vi "FlexibleBlock - Finite PCM Acquisition(Slave) - Left justified TI.vi"() -> ()   [LabVIEW 2021]
uses:
  <vilib>/PDM Acquisition Toolkit/host/Classes/Session/Controls/Logic Levels.ctl
  <vilib>/PDM Acquisition Toolkit/shared/controls/PCM Data Format Configuration.ctl
  <vilib>/PDM Acquisition Toolkit/shared/controls/Digital Edge.ctl
  <vilib>/PDM Acquisition Toolkit/shared/controls/PCM Bit Endianness.ctl
  <vilib>/PDM Acquisition Toolkit/shared/controls/PCM Data Justification.ctl
  <vilib>/PDM Acquisition Toolkit/shared/controls/PCM Frame Sync Control.ctl
  Program Files/National Instruments/LabVIEW 2021/examples/PDM Acquisition Toolkit/subVIs/PCM Interface Type.ctl
  Users/Admin/Desktop/Release audio branch/Audio/audio_d/audio_MeasurementService/source/measurements/ac/audio_acMeasurement/Measurement Results.ctl
  <vilib>/PDM Acquisition Toolkit/host/Classes/Tasks/PDM Tasks/Controls/Acquisition Mode.ctl
  <vilib>/addons/_NISVFA/_Shared subVIs/Controls/svc_Window.ctl
  <vilib>/addons/_NISVFA/_Shared subVIs/Common/SVL Set dB Reference (N Ch - 1 Ref).vi
  <vilib>/addons/Sound and Vibration/svt_Level/SVL AC & DC Level (Time) (N Ch).vi
  <vilib>/addons/Sound and Vibration/svt_Single Tone Measurements/SVT Spurious Free Dynamic Range (Frequency) (1 Ch).vi
  <vilib>/addons/_NISVFA/_Spectrum Processing/SVFA Unit Conversion (Complex) (1 Ch).vi
  <vilib>/addons/_NISVFA/_Shared subVIs/Common/SVL Set dB Reference (1 Ch).vi
  <vilib>/addons/Sound and Vibration/svt_Level/SVL AC & DC Level (Time) (1 Ch).vi
  <vilib>/addons/_NISVFA/_Spectrum Processing/SVFA Get Spectrum Subset.vi
  <vilib>/addons/_NISVFA/_Spectrum Processing/SVFA Get Spectrum Subset (Complex) (1 Ch).vi
  <vilib>/addons/_NISVFA/_Shared subVIs/Common/svc_Window Parameters.vi
  <vilib>/addons/_NISVFA/_Shared subVIs/Common/svc_Extract Single Tone Information (complex).vi
  <vilib>/addons/_NISVFA/_Shared subVIs/Common/svc_Check Frequency Range in Spectrum.vi
  <vilib>/addons/_NISVFA/_Spectrum Processing/SVFA Spectrum Peak Search.vi
  <vilib>/addons/_NISVFA/_Spectrum Processing/SVFA Spectrum Peak Search (1 Ch).vi
  <vilib>/addons/_NISVFA/_Shared subVIs/Common/svc_Spectrum Units.vi
  <vilib>/addons/_NISVFA/_Shared subVIs/Common/svc_Log View for Spectrum (1Ch).vi
  <vilib>/addons/_NISVFA/_Spectrum Processing/SVFA Unit Conversion (1 Ch).vi
  <vilib>/addons/_NISVFA/_Shared subVIs/Common/svc_Complex Datatype Defaults.vi
  <vilib>/addons/_NISVFA/_Shared subVIs/Common/svc_Build Unit Label for Frequency Range.vi
  <vilib>/addons/_NISVFA/_Shared subVIs/Common/SVL Set dB Reference (variant).vi
  <vilib>/addons/_NISVFA/_Shared subVIs/Common/svc_Get SV Channel Info.vi
  <vilib>/Analysis/baseanly.llb/Mean.vi
  <vilib>/Analysis/baseanly.llb/Mean (DBL).vi
  <vilib>/addons/_NISVFA/_Shared subVIs/Windowing/svfa_Scaled Time Domain Window (Array).vi
  <vilib>/addons/_NISVFA/_Spectrum Processing/SVFA Get Tone Amplitude and Phase (1 Ch).vi
  <vilib>/addons/_NISVFA/_Spectrum Processing/subVIs/svfa_Compute Complex Spectrum for Export.vi
  <vilib>/addons/_NISVFA/_Shared subVIs/Common/svc_Check Frequency Range in Bandwidth.vi
  <vilib>/addons/_NISVFA/_Shared subVIs/Common/svc_Convert Start and Stop to Start Index and Length.vi
  <vilib>/addons/_NISVFA/_Spectrum Processing/subVIs/svfa_Spectrum Peak Search.vi
  <vilib>/addons/_NISVFA/_Shared subVIs/Common/svc_Format Value (DBL).vi
  <vilib>/addons/_NISVFA/_Shared subVIs/Common/svc_Get Weighting Enum and Labels.vi
  <vilib>/addons/_NISVFA/_Shared subVIs/Common/svc_Engineering Units to Unit Label.vi
  <vilib>/addons/_NISVFA/_Shared subVIs/Common/svc_Surround NonAlpha String with Parentheses.vi
  <vilib>/dlg_ctls.llb/Space Constant.vi
  <vilib>/addons/_NISVFA/_Shared subVIs/Common/svc_Unwrap Phase.vi
  <vilib>/addons/_NISVFA/_Shared subVIs/Common/svc_Convert Spectrum Array to dB.vi
  <vilib>/addons/_NISVFA/_Spectrum Processing/subVIs/svfa_Conversion Utility (spectrum info).vi
  <vilib>/addons/_NISVFA/_Shared subVIs/Common/svc_Unit Label to Engineering Units.vi
  <vilib>/addons/_NISVFA/_Spectrum Processing/subVIs/svfa_Spectrum Info Window to windowTd Type Def.vi
  <vilib>/Analysis/4window.llb/Force Window.vi
  <vilib>/Analysis/4window.llb/Force Window (DBL).vi
  <vilib>/Analysis/4window.llb/Exponential Window.vi
  <vilib>/Analysis/4window.llb/Exponential Window (DBL).vi
  <vilib>/addons/_NISVFA/_Spectrum Processing/subVIs/svfa_Window Frequency Response.vi
  <vilib>/addons/_NISVFA/_Spectrum Processing/subVIs/svfa_Window Frequency Response (double array).vi
  <vilib>/Analysis/baseanly.llb/Dot Product.vi
  <vilib>/Analysis/baseanly.llb/Complex Dot Product.vi
  <vilib>/addons/_NISVFA/_Spectrum Processing/subVIs/svfa_Peak Rough Search Indices.vi
  <vilib>/addons/_NISVFA/_Shared subVIs/Common/svc_Unit Label Lexical Class.vi
  <vilib>/addons/_NISVFA/_Spectrum Processing/subVIs/svfa_Peak to RMS to Peak2Peak.vi
  <vilib>/addons/_NISVFA/_Spectrum Processing/subVIs/svfa_Mag to Mag2.vi
  <vilib>/addons/_NISVFA/_Spectrum Processing/subVIs/svfa_Linear to dB.vi
  <vilib>/addons/_NISVFA/_Spectrum Processing/subVIs/svfa_dBrefA to dBrefB.vi
  <vilib>/addons/_NISVFA/_Spectrum Processing/subVIs/svfa_Spectrum to Spectral Density.vi
  <vilib>/addons/_NISVFA/_Spectrum Processing/subVIs/svfa_Rect Window Frequency Response.vi
  <vilib>/addons/_NISVFA/_Spectrum Processing/subVIs/svfa_Cosine Window Coefficients.vi
  <vilib>/PDM Acquisition Toolkit/host/API/Public/Create Tasks/Create PCM Input Task.vi
  <vilib>/PDM Acquisition Toolkit/host/API/Public/Configure/Timing/Configure Timing - PCM Input Slave.vi
  <vilib>/PDM Acquisition Toolkit/host/API/Public/Configure/PDM Channel/Configure Microphone Sensitivity FSPA - PCM Input Task.vi
  <vilib>/PDM Acquisition Toolkit/host/API/Public/Utility/Configure Simulation Mode - PCM Input Task.vi
  <vilib>/PDM Acquisition Toolkit/host/API/Public/Start/Start PCM Input Task.vi
  <vilib>/PDM Acquisition Toolkit/host/API/Public/Read/Read PCM Input Waveform.vi
  <vilib>/measure/matone.llb/Extract Single Tone Information N Chan.vi
  <vilib>/PDM Acquisition Toolkit/host/API/Public/Clear/Clear PCM Input Task.vi
  <vilib>/addons/Sound and Vibration/svt_Weighting/SVT Weighting Filter (N Ch).vi
  <vilib>/addons/_NISVFA/_Shared subVIs/Common/svc_Caller VI Returned in Error Source.vi
  <vilib>/addons/_NISVFA/_Shared subVIs/Common/svc_Get Window Info.vi
  <vilib>/Analysis/0measdsp.llb/Scaled Time Domain Window.vi
  <vilib>/Analysis/0measdsp.llb/Scaled Time Domain Window (DBL).vi
  <vilib>/Utility/error.llb/Error Cluster From Error Code.vi
  <vilib>/Analysis/baseanly.llb/Std Deviation and Variance.vi
  <vilib>/addons/Sound and Vibration/svt_Single Tone Measurements/SVT Gain (Time) (1 Ch).vi
  <vilib>/addons/Sound and Vibration/svt_Distortion/SVT SNR without Harmonics (Frequency) (1 Ch).vi
  <vilib>/addons/Sound and Vibration/svt_Single Tone Measurements/SVT Dynamic Range (Frequency) (1 Ch).vi
  <vilib>/addons/Sound and Vibration/svt_Distortion/subVIs/sv_Check Data Valid (Audio) (1 Ch).vi
  <vilib>/addons/_NISVFA/_Shared subVIs/Common/svc_Convert Frequency to Frequency String.vi
  <vilib>/Analysis/4window.llb/window parameters.vi
  <vilib>/Analysis/4window.llb/Window Properties.vi
  <vilib>/Analysis/4window.llb/Window Properties by Name.vi
  <vilib>/addons/_NISVFA/_Spectrum Processing/subVIs/svfa_Spectrum Peak Tone Search and Estimation (complex).vi
  <vilib>/measure/masignal.llb/Tones and Noise Waveform.vi
  <vilib>/addons/_NISVFA/_Shared subVIs/Common/svc_FFT with Window.vi
  <vilib>/Analysis/1siggen.llb/Square Wave.vi
  <vilib>/addons/_NISVFA/_Spectrum Processing/subVIs/svfa_Three Finger Peak Search.vi
  <vilib>/addons/Sound and Vibration/svt_Distortion/subVIs/sv_Peak View Amplitude (1 Ch).vi
  <vilib>/PDM Acquisition Toolkit/host/API/PDM Acquisition Toolkit.lvlib
  <vilib>/PDM Acquisition Toolkit/host/Classes/Tasks/PDM Tasks/PDM Task.lvclass
  <vilib>/measure/NI_MAPro.lvlib
  <vilib>/PDM Acquisition Toolkit/shared/PDM Shared.lvlib
  <vilib>/addons/Sound and Vibration/svt_Single Tone Measurements/SoundVib_SingleTone.lvlib
  <vilib>/addons/Sound and Vibration/svt_Distortion/SoundVib_Distortion.lvlib
  <vilib>/addons/Sound and Vibration/svt_Weighting/SoundVib_ABCWeighting.lvlib
  <vilib>/PDM Acquisition Toolkit/host/Classes/Session/DecoderSession.lvclass
  Users/Admin/Desktop/Release audio branch/Audio/audio_d/audio_MeasurementService/source/measurements/ac/audio_acMeasurement/audio_acMeasurement.lvlib
panel:
  out "FreqDomainGraph":cluster{"x0":dbl, "dx":dbl, "magnitude":dbl[]}(graph) caption="AC"
  out "output cluster":T1
  out "error out 2":errorcluster
  in  "Latch Delay(ns)":sgl
  in  "PCM Interfaces":T2=enum."Left Justified"
  out "elements remaining":u32[](array[numeric])=[26]
  out "Frame Sync Clock Control":T3={"Frame Length"=64, "Frame Sync Pulse Width"=32, "Bit Clock Edge  Sync"=enum."Falling"}
  out "PCM Data Configuration":T5={"Frame Sync Edge for Channel 0"=enum."Falling", "Channel Count Per Frame"=2, "Channel Length"=32, "Bit Depth"=24, "Channel 0 Offset"=1, "Endianness"=enum."MSB First", "Data Justification"=enum."Left Justified"}
  in  "Bit clock rate":u32=12288000 format="%.4p"
  in  "logic level":T8
  out "Requested Sampling Rate":dbl=192000.0 format="%#_6p"
  out "detected phases (deg)":dbl[](array[numeric])=[48.77177137902379, 163.50683535190996] format="%.2p"
  out "detected amplitudes":dbl[](array[numeric])=[0.002127835538874218, 39.382575869286214] format="%.2p"
  out "detected frequencies":dbl[](array[numeric])=[87725.90443160792, 99.99819936214169] format="%.2p"
  in  "simulation mode":bool
  out "PCM Data":waveform(dbl)[](graph)=[{"t0"=timestamp(0 s since 1904-01-01), "dt"=5.208333277550992e-06, "Y"=array[4000 elements], "attributes"=variant("NI_ChannelName"=variant(string "PCMI0.0"))}, {"t0"=timestamp(0 s since 1904-01-01), "dt"=5.208333277550992e-06, "Y"=array[4000 elements], "attributes"=variant("NI_ChannelName"=variant(string "PCMI0.1"))}]
  in  "microphone sensitivity (dB/Pa)":dbl=0.34762
  in  "number of words":i32=19200
  in  "channel list":string="7820\\PCMi 0"
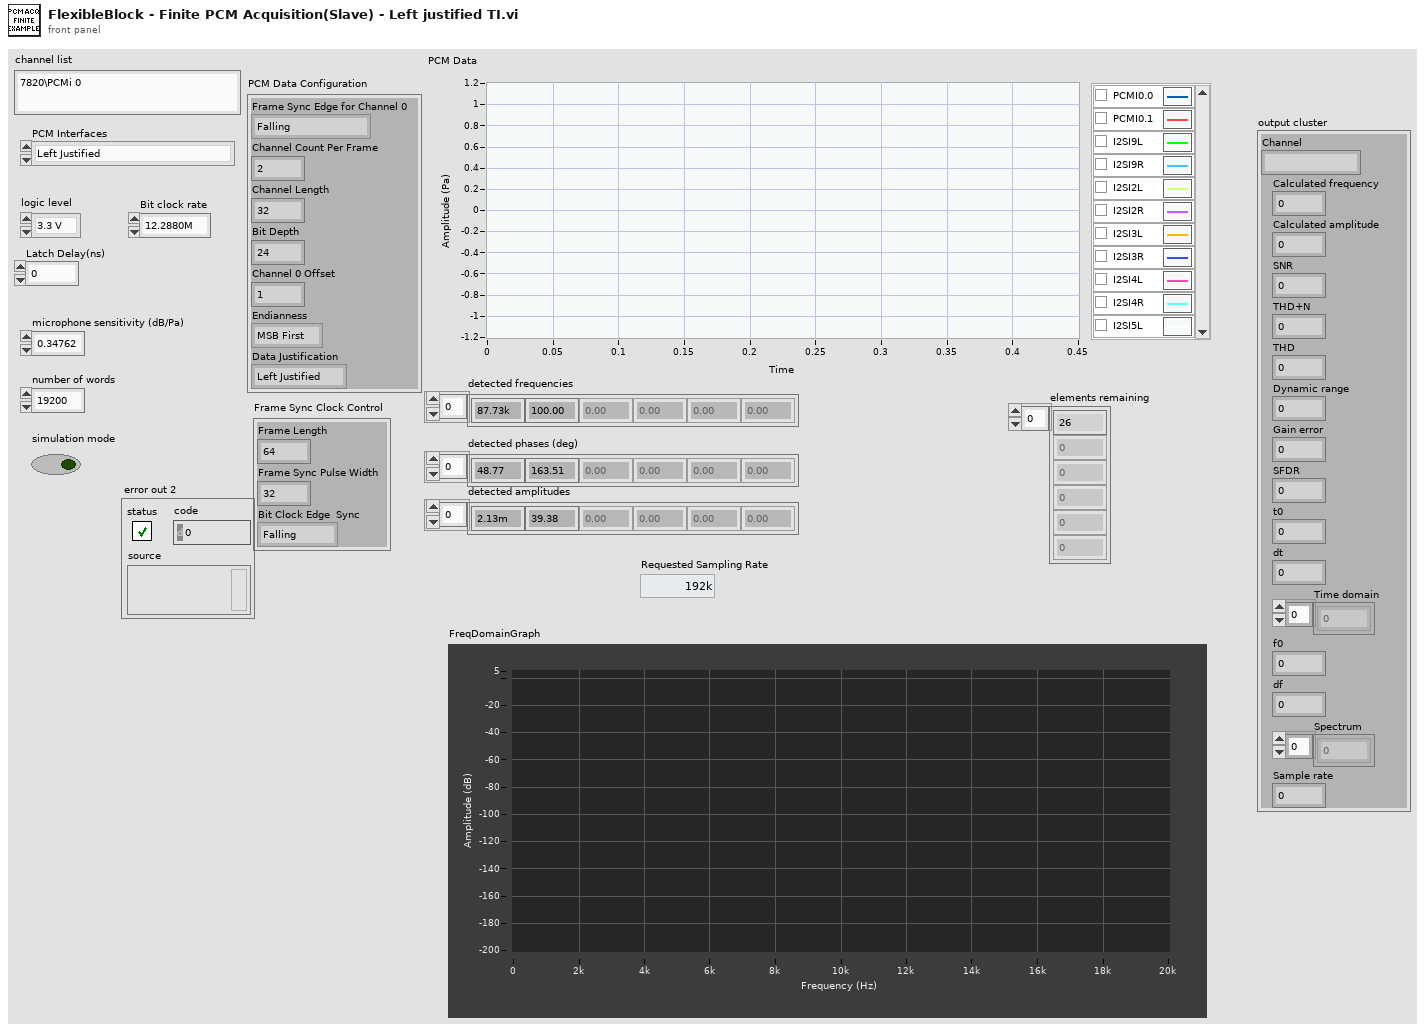
[diagram p1: front panel]
types:
  T1 = typedef "audio_acMeasurement.lvlib/Measurement Results.ctl" = cluster{"Channel":string, "Calculated frequency":dbl, "Calculated amplitude":dbl, "SNR":dbl, "THD+N":dbl, "THD":dbl, "Dynamic range":dbl, "Gain error":dbl, "SFDR":dbl, "t0":dbl, "dt":dbl, "Time domain":dbl[], "f0":dbl, "df":dbl, "Spectrum":dbl[], "Sample rate":u32}
  T2 = typedef "PCM Interface Type.ctl" = enum16{"I2S", "Left Justified", "Right Justified", "TDM 4 Channel", "TDM 6 Channel", "TDM 8 Channel", "DSP mode", "DSP mode with 1 bit delay", "PCM Short Frame", "PCM Long Frame"}
  T3 = typedef "PDM Shared.lvlib/PCM Frame Sync Control.ctl" = cluster{"Frame Length":u16, "Frame Sync Pulse Width":u16, "Bit Clock Edge  Sync":T4}
  T4 = typedef "PDM Shared.lvlib/Digital Edge.ctl" = enum8{"Rising", "Falling"}
  T5 = typedef "PDM Shared.lvlib/PCM Data Format Configuration.ctl" = cluster{"Frame Sync Edge for Channel 0":T4, "Channel Count Per Frame":u8, "Channel Length":u16, "Bit Depth":u8, "Channel 0 Offset":u16, "Endianness":T6, "Data Justification":T7}
  T6 = typedef "PDM Shared.lvlib/PCM Bit Endianness.ctl" = enum16{"MSB First", "LSB First"}
  T7 = typedef "PDM Shared.lvlib/PCM Data Justification.ctl" = enum16{"Left Justified", "Right Justified"}
  T8 = typedef "PDM Acquisition Class Library.lvlib/DecoderSession.lvclass/Logic Levels.ctl" = enum16{"3.3 V", "1.8 V", "1.2 V"}
  T9 = cluster{"Channel":string, "Calculated frequency":dbl, "Calculated amplitude":dbl, "SNR":dbl, "THD+N":dbl, "THD":dbl, "Dynamic range":dbl, "Gain error":dbl, "SFDR":dbl, "t0":dbl, "dt":dbl, "Time domain":dbl[], "f0":dbl, "df":dbl, "Spectrum":dbl[], "Sample rate":u32}
  T10 = cluster{"start frequency":dbl, "stop frequency":dbl}
  T11 = enum16{"no change", "spectrum", "spectral density"}
  T12 = cluster{"linear/dB":enum16{"no change", "linear", "dB"}, "dB reference (0: no change)":dbl, "power/magnitude":enum16{"no change", "power", "magnitude"}, "view":enum16{"no change", "rms", "peak", "peak-peak"}}
  T13 = cluster{"gain units":enum16{"dB", "linear ratio"}, "detected fundamental amplitude units":enum16{"EU rms", "EU peak", "EU peak-peak"}}
  T14 = typedef "svc_Window.ctl" = u32
  T15 = cluster{"SNR units":enum16{"dB", "linear ratio", "%"}, "detected fundamental amplitude units":enum16{"EU rms", "EU peak", "EU peak-peak"}}
  T16 = typedef "PDM Acquisition Class Library.lvlib/PDM Task.lvclass/Acquisition Mode.ctl" = enum16{"Finite", "Continuous"}
  T17 = typedef "PDM Acquisition Class Library.lvlib/PCM Input Task.lvclass/DVR PCM Input Task.ctl" = refnum<data-value>
  T18 = typedef "svc_Spectrum Info.ctl" = cluster{"channel name":string, "description":string, "x-axis units":T19, "spectral info":cluster{"spectrum type":T20, "linear/dB":enum16{"linear", "dB"}, "window":u16, "window size":i32, "FFT size":i32}, "engineering units":T21, "custom label":string, "dB reference [EU]":dbl, "peak units":enum16{"rms", "peak", "peak-peak"}, "weighting filter":T22, "spectral density?":bool, "unit label":string, "spectrum skewed?":bool, "complimentary spectrum units":T23}
  T19 = typedef "svc_X-Axis Units.ctl" = u16
  T20 = typedef "svc_Spectrum Type.ctl" = enum16{"FFT Spectrum [complex]", "Amplitude [Magnitude]", "Power [Magnitude^2]", "Cross Spectrum [complex]", "Frequency Response [Complex]"}
  T21 = typedef "svc_Engineering Units Text Ring.ctl" = u16
  T22 = typedef "svc_Weighting Filter Text Ring.ctl" = u16
  T23 = typedef "svc_Complimentary Spectrum Units.ctl" = enum16{"none", "radians", "degrees", "cycles", "imaginary"}
  T24 = cluster{"complex spectrum response":cluster{"f0":dbl, "df":dbl, "complex spectrum":cdb[]}, "spectrum info":T18}
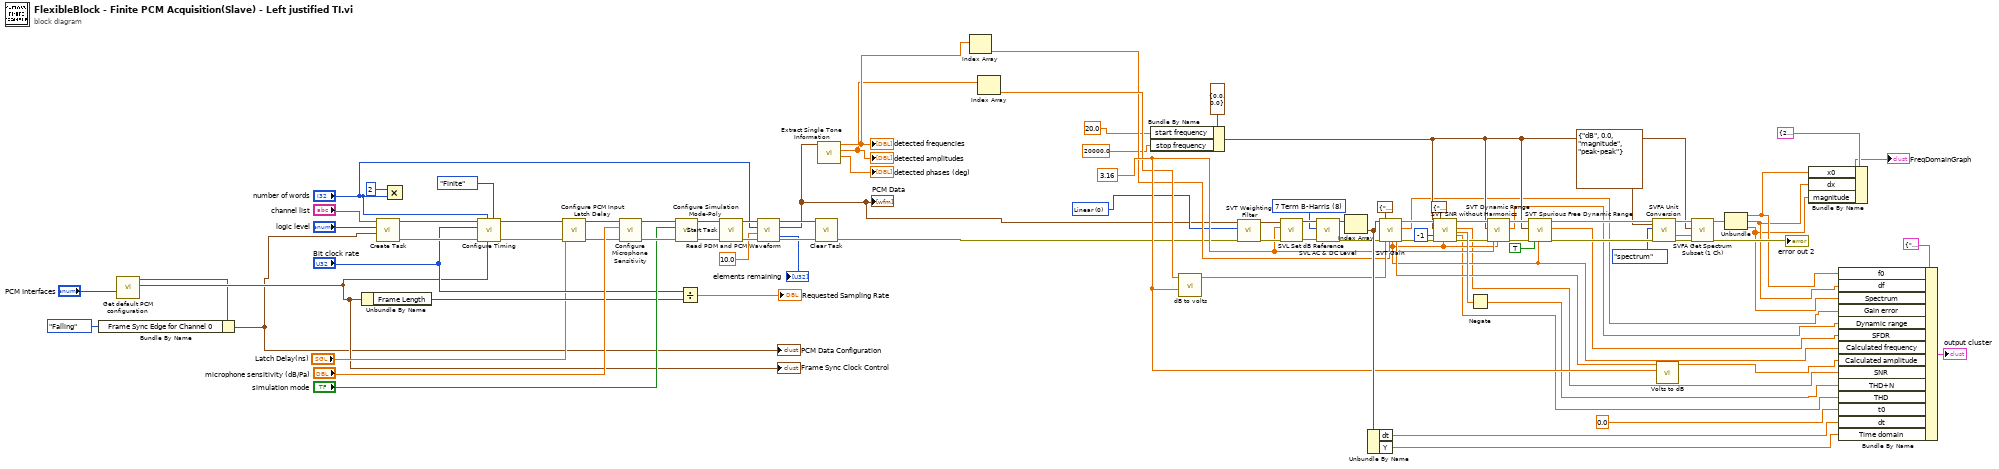
[diagram p0: block diagram]
diagram:
  w25 = u16 0 items=["Linear", "A-weighting", "B-weighting", "C-weighting"] ("weighting")
  w28 = 3.16 ("start frequency")
  w44 = T14 8 items=["None"=0, "Hanning"=1, "Hamming"=2, "Blackman-Harris"=3, "Exact Blackman"=4, "Blackman"=5, "Flat Top"=6, "4 Term B-Harris "=7, "7 Term B-Harris"=8, "Low Sidelobe"=9, "Force"=64, "Exponential"=65, "Blackman Nuttall"=11, "Triangle"=30, "Bartlett-Hanning"=31, "Bohman"=32, "Parzen"=33, "Welch"=34, "Kaiser"=60, "Dolph-Chebyshev"=61, "Gaussian"=62] ("window")
  n1 = call "Get default PCM configuration.vi"("PCM Interfaces"="PCM Interfaces") -> ("Frame Sync Clock Control"=w64:T3, "PCM Data Configuration"=w63:T5)  [unwired: 9 in]
  "Frame Sync Clock Control" <- w64
  n2 = Bundle By Name(cluster=w63, "Frame Sync Edge for Channel 0"=Digital_Edge."Falling") -> (w62:T5)
  "PCM Data Configuration" <- w62
  n3 = Unbundle By Name(w64) -> ("Frame Length"=w70:u16)
  n4 = call-poly <vilib>:"Create Task.vi"("PCM data configuration"=w62, "logic level"="logic level", "channel list"="channel list") -> ("error out"=w81:errorcluster, "PCM input task out"=w80:T17)  [unwired: 7 in]
  n5 = Multiply(x=2, y="number of words") -> ()  [unwired: 1 out]
  n6 = call-poly <vilib>:"Configure Timing.vi"("acquisition mode"=Acquisition_Mode."Finite", "Frame Sync Clock Control"=w64, "number of words per channel"="number of words", "error in"=w81, "Bit Clock rate"="Bit clock rate", "PCM input task in"=w80) -> ("error out"=w79:errorcluster, "PCM input task out"=w72:T17)  [unwired: 4 in]
  n7 = call <vilib>:"Configure PCM Input Latch Delay.vi"("error in"=w79, "Latch Delay(ns)"="Latch Delay(ns)", "PCM input task in"=w72) -> ("error out"=w78:errorcluster, "PCM input task out"=w77:T17)  [unwired: 6 in, 1 out]
  n8 = call-poly <vilib>:"Configure Microphone Sensitivity.vi"("error in"=w78, "microphone sensitivity (FS/Pa)"="microphone sensitivity (dB/Pa)", "PCM input task in"=w77) -> ("error out"=w85:errorcluster, "PCM input task out"=w84:T17)  [unwired: 7 in]
  n9 = call-poly <vilib>:"Configure Simulation Mode-Poly.vi"("error in"=w85, "simulation mode"="simulation mode", "PCM Input Task in"=w84) -> ("error out"=w75:errorcluster, "PCM Input Task out"=w76:T17)  [unwired: 7 in]
  n10 = Divide(x="Bit clock rate", y=w70) -> (x/y=→"Requested Sampling Rate":dbl)
  n11 = call-poly <vilib>:"Start Task.vi"("error in"=w75, "PCM input task in"=w76) -> ("error out"=w89:errorcluster, "PCM input task out"=w88:T17)  [unwired: 8 in]
  n12 = call-poly <vilib>:"Read PDM and PCM Waveform.vi"("error in"=w89, "timeout"=10.0, "words per channel"="number of words", "PCM input task In"=w88) -> ("error out"=w87:errorcluster, "PCM waveforms"=w8:waveform(dbl)[], "PCM input task out"=w86:T17, "elements remaining"=→"elements remaining":u32[])  [unwired: 4 in]
  "PCM Data" <- w8
  n13 = call-poly <vilib>:"Clear Task.vi"("error in"=w87, "PCM input task in"=w86) -> ("error out"=w9:errorcluster)  [unwired: 9 in]
  n14 = call-poly <vilib>:"Extract Single Tone Information.vi"("time signals in"=w8) -> ("detected phases (deg)"=→"detected phases (deg)":dbl[], "detected amplitudes"=w6:dbl[], "detected frequencies"=w7:dbl[])  [unwired: 5 in, 3 out]
  "detected frequencies" <- w7
  "detected amplitudes" <- w6
  n15 = Index Array(array=w7) -> (element=w26:dbl)  [unwired: 1 in]
  n16 = Index Array(array=w6) -> (element=w27:dbl)  [unwired: 1 in]
  n17 = Bundle By Name(cluster=T10 {"start frequency"=0.0, "stop frequency"=0.0} ("frequency range"), "start frequency"=20.0, "stop frequency"=20000.0 ("start frequency")) -> (w33:T10)
  n18 = call "dB to volts.vi"("Full scale range"=w28, "Voltage(dB)"=w27) -> ("Voltage(volts)"=w37:dbl)  [unwired: 9 in]
  n19 = call-poly <vilib>:"SVT Weighting Filter.vi"("error in (no error)"=w9, "weighting"=w25, "scaled signals [EU]"=w8) -> ("error out"=w58:errorcluster, "weighted signals [EU]"=w57:waveform(dbl)[])  [unwired: 6 in]
  n20 = call-poly <vilib>:"SVL Set dB Reference.vi"("error in (no error)"=w58, "dB reference [EU]"=w28, "scaled signals in [EU]"=w57) -> ("error out"=w45:errorcluster, "scaled signals out [EU]"=w47:waveform(dbl)[])  [unwired: 7 in]
  n21 = call-poly <vilib>:"SVL AC & DC Level.vi"("scaled signals in [EU]"=w47, "window"=w44, "error in (no error)"=w45) -> ("AC signals [EU]"=w46:waveform(dbl)[], "error out"=w53:errorcluster)  [unwired: 11 in, 4 out]
  n22 = Index Array(array=w46) -> (element=w60:waveform(dbl))  [unwired: 1 in]
  n23 = Unbundle By Name(w60) -> ("dt"=w15:dbl, "Y"=w14:dbl[])
  n24 = call-poly <vilib>:"SVT Gain.vi"("scaled signal [EU]"=w60, "error in (no error)"=w53, "desired units"=T13 {"gain units"=enum."dB", "detected fundamental amplitude units"=enum."EU peak"}, "amplitude [EU peak]"=w37, "expected fundamental frequency [Hz]"=w26) -> ("detected fundamental\nfrequency [Hz]"=w21:dbl, "detected fundamental\namplitude"=w36:dbl, "complex spectrum"=w42:T24, "gain"=w24:dbl, "error out"=w43:errorcluster)  [unwired: 9 in, 1 out]
  n25 = call-poly <vilib>:"SVT SNR without Harmonics.vi"("complex spectrum"=w42, "frequency range"=w33, "maximum harmonic"=-1, "error in (no error)"=w43, "desired units"=T15 {"SNR units"=enum."dB", "detected fundamental amplitude units"=enum."EU rms"}, "expected fundamental frequency [Hz]"=w21) -> ("complex spectrum"=w49:T24, "SNR (without harmonics)"=w19:dbl, "SINAD"=w50:dbl, "THD"=w17:dbl, "error out"=w48:errorcluster)  [unwired: 6 in, 3 out]
  n26 = Negate(x=w50) -> (-x=w18:dbl)
  n27 = call-poly <vilib>:"SVT Dynamic Range.vi"("complex spectrum"=w49, "frequency range"=w33, "error in (no error)"=w48, "full scale amplitude [EU peak]"=w28, "expected fundamental\nfrequency [Hz]"=w21) -> ("dup complex spectrum"=w54:T24, "dynamic range"=w23:dbl, "error out"=w55:errorcluster)  [unwired: 9 in, 3 out]
  n28 = call-poly <vilib>:"SVT Spurious Free Dynamic Range.vi"("complex spectrum"=w54, "frequency range"=w33, "error in (no error)"=w55, "exclude harmonics"=TRUE, "expected fundamental\nfrequency [Hz]"=w21) -> ("complex spectrum"=w40:T24, "spurious free dynamic range"=w22:dbl, "error out"=w41:errorcluster)  [unwired: 7 in, 5 out]
  n29 = call-poly <vilib>:"SVFA Unit Conversion.vi"("complex spectrum"=w40, "desired scaling"=T12 {"linear/dB"=enum."dB", "dB reference (0: no change)"=0.0, "power/magnitude"=enum."magnitude", "view"=enum."peak-peak"}, "spectral density desired"=T11."spectrum", "error in (no error)"=w41) -> ("converted spectrum"=w34:cluster{"x0":dbl, "dx":dbl, "magnitude":dbl[]}, "spectrum info out"=w30:T18, "error out"=w29:errorcluster)  [unwired: 10 in, 3 out]
  n30 = call "Volts to dB.vi"("Full scale range"=w28, "Voltage(V)"=w36) -> ("Voltage(dB)"=w20:dbl)  [unwired: 9 in]
  n31 = call <vilib>:"SVFA Get Spectrum Subset (1 Ch).vi"("spectrum"=w34, "range"=w33, "spectrum info"=w30, "error in (no error)"=w29) -> ("spectrum subset"=w32:cluster{"x0":dbl, "dx":dbl, "magnitude":dbl[]}, "error out"=→"error out 2":errorcluster)  [unwired: 10 in, 4 out]
  n32 = Unbundle(w32) -> ("x0"=w3:dbl, "dx"=w2:dbl, "magnitude"=w1:dbl[])
  n33 = Bundle By Name(cluster=cluster{"x0":dbl, "dx":dbl, "magnitude":dbl[]} {"x0"=20.000000214204196, "dx"=10.000000107102098, "magnitude"=[-114.15651603320237, -121.36305665533368, -143.37588801995145, -125.3747624869788, -122.11025021298603, -123.1180823220903, -136.70897783052968, -126.77027917479111, -124.020905313897, -126.88391294043589, -126.3843168978061, -126.4615231354403, -89.75481804806032, -54.76170840557006, -31.889535533022606, -16.187220558881673, -5.794808006347515, 0.16644842981875596, 2.111954876706231, 0.16568271315306057, -5.796393407051838, -16.18976327759025, -31.89341764484416, -54.76929643271966, -89.79463483193392, -125.27421120596713, -124.60058186076871, -123.95053059271027, -127.47180140959146, -139.09403229507976, -126.63006434840091, -121.07579620021035, -120.04129048879442, -123.47329398145577, -134.14891446501707, -146.20339758492725, -137.3896104617882, -126.31513036563122, -122.54359675626772, -122.43160900789394, -125.49078542917715, -130.19044820464535, -126.59317929836668, -124.64241946975281, -126.2021713620974, -128.1063542477712, -127.48703106495057, -125.76364372674362, -124.47688387334786, -125.23916835138252, -128.6971630825081, -136.56790005708194, -133.32615372072206, -131.72608576345402, -143.106858163413, -131.3095735071133, -124.29397195200927, -121.368674373711, -121.90246299165194, -128.19433975069393, -131.60782712391435, -126.8944252740466, -127.39742985708364, -127.71417117512829, -126.30679240498324, -125.19252731229923, -125.49993468715164, -126.39994800524063, -125.34042088344107, -124.67793859086814, -127.23965579624198, -135.84083632259842, -142.43150809477874, -134.0086167972518, -130.73012726416758, -130.1907568018264, -135.50609265421332, -133.4253285970364, -129.60229987874516, -131.13171834262775, -133.59386870323485, -135.71425492413542, -142.2170082364512, -136.95982490530557, -129.38136777852714, -127.98134492981278, -129.6797996357936, -130.20168657208524, -129.69250116743794, -132.18606004254426, -139.3365319883325, -142.95638009021565, -140.10103077135625, -137.90125131233873, -138.1172575189856, -137.12270326430053, -134.75157359049484, -131.036141399244, -129.58819028859088, -132.3121381683547, -132.23899142800224, -129.61404290235913, -131.74863783055739, -134.97852492231073, -130.67217091078922, -129.57964087194782, -130.57762641281138, -132.52834075522017, -135.78627621884178, -142.49901499322274, -141.48800399558812, -143.24757389814621, -136.19253726244997, -126.53142536309788, -123.34303583389666, -123.21233963987521, -124.41973762027126, -125.22134897615948, -126.9196904339552, -134.53612798046296, -131.3511435877546, -125.7114183660295, -126.40782929669791, -130.9162950852669, -131.9594582891918, -129.02418942942936, -127.10971294232291, -126.4224310677424, -126.82612865454529, -127.28676420603188, -126.88338795412825, -125.99706987988446, -125.40605453150732, -125.98578839299827, -127.64455962189358, -129.75927585242462, -133.09905622646616, -135.7466207774017, -134.00685547109643, -132.67495090714914, -132.22911014695032, -134.46516716691167, -132.93107087889965, -129.16213188426514, -128.36475477295505, -130.6578239989015, -139.01319588309485, -141.43076278882998, -132.5976905198517, -130.20172638885097, -131.94249777520935, -142.4683868052605, -137.91371427959592, -134.69530409837475, -139.30771283308204, -143.64947826069582, -132.63466050522175, -128.7962369961467, -128.39937836768866, -131.74873055308265, -138.6954450934956, -135.1962285419425, -132.09709522748193, -129.15949687453383, -126.11694756949157, -124.63202529768226, -124.94201741482676, -126.49196300473305, -128.6821678936123, -130.15958004607992, -130.1273796587127, -128.5745132662968, -128.1058374455199, -127.97528167034748, -126.56114707595619, -125.96083493714872, -128.04071224807072, -133.1177878962448, -133.10886671363295, -130.02517062749695, -127.71565199687112, -126.283155806085, -125.27620474949131, -124.43103341153218, -125.55086008570059, -127.69603922360118, -124.9973939221027, -123.63561955277645, -126.02696667962155, -131.0339686597125, -130.35947614827558, -128.56581326055817, -129.36696386233123, -131.51058997650355, -131.49345793307128, -130.2639756951258, -130.06154137992266, -131.30934831123636, -133.68725043425223, -131.21024897603903, -127.41427463637223, -126.56702895822193, -128.73574657204506, -135.2251528562724, -137.09878796045234, -129.65982047361766, -128.60824269595017, -133.9629685197531, -143.45429853804876, -133.13793023312388, -136.3576930963645, -140.18866650698027, -136.62431834777468, -149.51000061331155, -138.2575481284217, -135.40077239669253, -133.70402963095603, -129.62130848019223, -128.04003889661385, -129.07299362960455, -130.243010381597, -130.8356545145397, -134.25554995048782, -142.81225234393412, -143.35431562967096, -141.99768795418544, -133.72891879653776, -128.26376229949614, -126.4404753422564, -127.664694958722, -131.6546151781298, -133.9835508288192, -131.61025037102488, -129.76355892054818, -129.2146948095566, -130.47903981575715, -130.70294733784036, -127.96757949868831, -126.35288406579076, -126.31353409151642, -127.69465408451497, -130.10696674453473, -133.9953538092625, -138.95937651820464, -134.78023022337968, -133.40331646844584, -136.97210669828902, -137.6742245731884, -131.8935865116608, -128.08041416654765, -126.6030376158959, -129.1229728616486, -136.23524607274658, -137.99763315178393, -137.663888314118, -132.81444112514913, -128.94913192656026, -127.91873209867715, -128.83649192854074, -131.96946924832557, -140.50334657728865, -139.17357143500712, -130.04685541139634, -127.55399107211304, -128.5346865441011, -130.05619208428828, -131.5359224551727, -135.30272276609026, -140.56598466588264, -137.53864581132396, -135.36650264777796, -132.05021553801907, -127.08431322796868, -125.11638153620895, -126.51546380508822, -130.79487082356053, -135.8337500700424, -137.96789098268383, -137.6612174967581, -136.8525240136817, -137.89560180300387, -138.4163606363077, -138.89617197328573, -151.05555360581963, -140.0806379283803, -133.13438691626533, -130.67742331158985, -132.7009758726239, -137.7930300440105, -133.89079268203173, -132.3513933225086, -129.47466790985249, -128.675174172983, -134.2508781117415, -144.38217949112027, -143.25302137407414, -138.2432387296004, -133.18816048984561, -132.4476521016706, -132.27940648212274, -133.71593106085697, -130.97272419663955, -128.0071750015209, -128.32320844829786, -128.1322204714087, -126.11314825211852, -124.75764507735195, -125.00183660902866, -126.3881992622004, -126.68597521000366, -126.47721627454001, -128.63325217073626, -133.5154813873756, -133.6547303137009, -130.43733361296495, -127.71962150682313, -126.65473252724156, -128.18456744976507, -132.61617788973518, -138.6744162847475, -136.89280772607157, -131.05936965553266, -127.65982792402667, -127.61911554281396, -132.6356704141472, -145.5088139707351, -133.11481581885226, -129.8172964765464, -127.96031242256109, -127.1624773550662, -127.5334945461254, -128.77045709086252, -130.75805320448512, -133.73785033851098, -137.40393383108562, -140.64919530242383, -139.86263481002896, -139.27568424715585, -139.3165680812446, -136.37848592977173, -131.85564512858738, -128.04553654018565, -127.10046843375338, -127.70132337470984, -129.95972346253058, -136.15651152512513, -151.45234338455992, -136.34769248734867, -129.85335842932597, -125.62043839550992, -124.93110634255333, -127.2719922492762, -131.50099109954363, -134.24251753241893, -133.64061920992432, -135.34907730259997, -136.9361750228094, -139.4942004419679, -138.71830754900066, -131.35348239280097, -129.1847565855113, -128.93742401816604, -130.19230746987208, -132.7003727659455, -133.0516777985375, -130.97536944584454, -129.80754972375604, -130.85995618012333, -134.60541803793487, -144.58433965498182, -141.48074325063288, -133.1142287798377, -129.33650564449522, -126.52083915451094, -124.85767547811555, -125.039205853284, -125.76775672688633, -124.84425555853855, -123.0842008695624, -122.65967897754992, -124.43434703908707, -127.94012361622373, -132.03180970270643, -134.74422956385382, -134.1429029523909, -133.170624676105, -130.4381023904983, -128.38182637668285, -127.11788204516643, -126.09625608617152, -125.73095172423793, -126.56078991113168, -130.53076936926968, -147.6711161082625, -134.73874285097045, -132.45010923546954, -139.20610994728972, -144.12038561407957, -139.2934665775726, -133.33941953498666, -133.87196938118532, -137.92251592965744, -134.54376376378838, -135.10465774938206, -138.00036784453525, -140.14923829069366, -140.73594612300715, -135.31978861803103, -137.74981196351, -138.26679599379776, -130.02808759228776, -128.26232136313172, -129.5641718920475, -132.19935058576607, -136.61513212940693, -137.70405663224665, -132.94970694747306, -131.44414608568366, -131.39825444499925, -129.0592354923359, -126.77224109121286, -126.35431094572881, -127.11920218331377, -128.1590380561889, -132.54602468036273, -147.4097457828696, -132.66405562662808, -130.71098010220967, -131.13083905442704, -134.78108336536906, -144.53443589755935, -135.07906733275942, -131.00735560209276, -129.39549573091338, -130.94279831223741, -135.41063782985458, -139.89715600727968, -136.8353301788793, -133.1637671688385, -132.53876951223558, -135.86101805382629, -133.90049747804736, -129.27812427844404, -127.35043485949639, -126.70321117078687, -127.45904928107025, -129.31783333493055, -129.92679474398406, -129.27971386920967, -130.00018536685386, -128.9859740832338, -127.74720161522279, -131.35885053377064, -148.81785299198384, -135.1841137130214, -131.30044601743242, -130.2603569676074, -130.8089224292011, -132.2498404542057, -133.65829608602294, -135.33263985349686, -131.89623349713796, -127.83325622000918, -127.22791275050872, -129.57278397746532, -133.40149275610327, -134.0800544187885, -131.9310482478005, -132.35412217024768, -138.58371220502386, -131.04898036877447, -126.62984506457768, -125.65832818838884, -126.79449295419846, -129.1989464618408, -128.89501813476937, -127.71055226666991, -128.35201039176778, -128.78196491305584, -127.67883831390327, -126.61656217913246, -127.21217342691894, -128.53623925730813, -127.68098815225079, -127.88852615448995, -128.4140889308591, -127.15131844869303, -125.61051516912214, -124.43626065305368, -125.2051776368406, -129.521146725487, -136.46092559983086, -133.9930073209309, -133.4073275429007, -144.590380697332, -134.34271862706476, -129.57012341874486, -130.00992420856122, -133.73251748553523, -141.5502231794172, -140.04976832277276, -134.5079774386407, -131.67807173506742, -130.4172360660502, -129.42565663046753, -128.92218492602433, -130.59264886399205, -133.7369795995416, -130.41321499027114, -128.31516713641906, -130.24025121906206, -137.12637454195058, -145.21921974900937, -134.7715825912015, -131.23532439184356, -130.2829285815037, -129.7996696612736, -131.59985598104026, -137.39979799305587, -145.93688668306794, -137.00808684890555, -130.6964697519213, -128.99477114198365, -129.31059962430828, -129.1301276791428, -128.50071981657925, -127.88315655628146, -126.46125341801414, -125.53895633397144, -126.10664095039637, -128.57319122135647, -129.87075018141476, -129.64489172570515, -132.56487087993452, -141.6528124552129, -139.24493094304057, -131.8661976364603, -129.48357920444943, -128.838194919264, -128.86696820719897, -129.1182549107291, -129.276752155319, -130.50307398251564, -131.99953643570313, -133.23539632489323, -138.4905558435136, -137.08561310159223, -131.39620717185255, -129.2081990042275, -129.10928031059265, -131.22866296683628, -132.52532548394962, -129.16741984258266, -127.162610480911, -129.75500709172277, -138.05884875708298, -132.22950034834076, -128.98504167735345, -126.62201834882076, -126.60869755269948, -129.88482749687927, -136.36335481024477, -136.13049587489897, -133.8884618323441, -130.84390588685744, -127.09543624684672, -126.45898289944327, -130.26337052071307, -132.27768221924157, -126.69271310562154, -124.77324115553408, -125.07700001103174, -126.39423779383688, -128.45690525550663, -132.88581266275648, -141.63160035134737, -131.6789666347667, -128.17411609759813, -127.86393006040691, -129.09857776095288, -130.37683399418086, -130.48857325472878, -131.97120435437375, -132.17255321428806, -128.82835770307037, -125.51831606305548, -123.74257230980672, -124.01121775813436, -127.3178662591301, -135.66201835184535, -132.2764362005697, -127.88921506195166, -126.49793506836055, -126.54317231546797, -128.28991369920078, -132.28041101886913, -134.36951957288161, -131.12640145365083, -130.53958667504926, -133.19516620998962, -140.0012901923717, -141.94929210952708, -136.07051703087043, -136.97684034414075, -140.00144181656984, -138.21612577381376, -140.76837369696437, -135.97989944881246, -133.01488465136433, -135.74568686311724, -138.4317533132987, -133.699313169655, -132.4857861537641, -131.70064319055524, -129.52009624293703, -127.02717936923707, -126.13225053347067, -127.68835165412906, -131.28683149164067, -132.793748900352, -133.70138952533594, -133.8150620263195, -130.51346391520588, -128.84985757832328, -127.68718694870275, -126.13638519540808, -125.27597045706825, -125.12895012765941, -125.20089966751287, -125.96008249177302, -128.0865349903974, -131.10087328748972, -134.75057982525985, -133.75328927395412, -130.45539097090005, -131.3194658841701, -141.90359796485697, -132.31741787919046, -126.8976040873404, -127.09010857421609, -131.01364642141783, -132.5608588172204, -133.1003527631429, -133.29649981808484, -129.55841592288726, -128.72567394837557, -132.45273358509388, -149.84866149457767, -137.67276113570475, -135.37470909323818, -140.12502387674152, -140.65755931138963, -130.09019903413676, -125.31903068060751, -123.44159833636911, -124.07844165525175, -126.27532781551463, -128.11698626517995, -129.93503279161055, -131.00534012754505, -130.16009147564688, -129.71748332913967, -131.20476346088725, -135.0606166107994, -138.21203916558733, -132.7377616824591, -129.9345422966717, -128.54500865501154, -127.00241898048121, -126.22443434895482, -126.61490509228963, -127.56257611580777, -129.39942205378213, -134.03174882812462, -135.55004397449244, -129.9464625852486, -127.00529096573051, -126.34429137874328, -127.802644811231, -129.71233311779847, -130.77955552504602, -134.11824341731727, -145.29073872325128, -130.86874952497348, -126.49219125362087, -125.51681287261788, -126.67449358683199, -129.02771456133084, -129.3818490067665, -128.51134286587535, -128.35620607495213, -128.11722401348587, -128.3130759548645, -129.99536595996952, -132.29064435013981, -130.70414529104724, -127.10006059467828, -125.70174942765972, -126.85029458207892, -130.05831133701048, -133.94553912926082, -140.0791993172447, -137.2780369565474, -133.1110770272686, -130.59818142231066, -126.9481921470033, -125.42892293135063, -125.4687758796935, -127.1641244302916, -132.98222674979925, -138.9734289321744, -131.49285227286728, -128.7694265812654, -127.73023640566508, -129.26444713524572, -135.16014944866103, -134.92392269671907, -132.9869975924077, -132.6795931101827, -132.04575219482038, -131.06532995620464, -129.8050719377489, -128.7406509520967, -130.3111202664169, -141.7229618143493, -132.8277450492622, -130.21071064893025, -134.62590313714688, -147.6384379221752, -138.7819109391997, -135.52537884096105, -141.51928967709938, -139.4185570167782, -137.57557999929907, -139.54572045143098, -137.68651212869054, -133.9467959834045, -134.1604389388604, -138.55688137983648, -131.525531225989, -127.22042353812448, -126.98616874013584, -129.3992002956473, -133.3532631917223, -133.70540902612575, -128.00339883058052, -125.39409563073635, -126.21233400228485, -128.75457392554503, -127.07712950709366, -126.11135063391721, -128.79979095374705, -133.70129910129313, -133.39740602632497, -132.31882383172749, -133.70939703773558, -137.90095688770901, -137.702406748392, -132.81796747938506, -130.18046750876536, -130.60775525183064, -132.62311309117305, -133.34982444438825, -133.5130876057437, -132.08906184840237, -129.8330907049975, -129.58934674394956, -130.7793666265536, -129.3312651115063, -129.00815038846991, -131.7868493277033, -136.15506251920868, -136.58953561343742, -136.98648329762946, -156.09154258422765, -136.3993207154312, -133.99911977430864, -134.5342642454817, -131.64377042290658, -129.28528970315546, -130.73713871730166, -138.1450242269703, -143.12771377142388, -135.5095193027515, -133.2827418379652, -133.78200524612797, -128.90434266259803, -125.47905925595104, -124.7851928330207, -126.98439231485304, -132.9594053683025, -136.9240663579998, -129.9024175644099, -125.317739570323, -123.6267210650635, -124.43267769156253, -127.37067687006046, -129.41517108910898, -129.20164631430853, -128.86899661862498, -128.11815230821324, -128.2115034976673, -129.53942198882626, -132.53444686451263, -143.4477692136308, -136.67568534681155, -130.90682944841578, -130.258104371618, -133.06896289787474, -145.39868164901216, -138.53183084544116, -134.50980778823376, -136.85875097828932, -140.61844640654363, -140.31205962196015, -133.8107222956887, -130.6110971462344, -131.87976429464007, -144.90403424309747, -132.20039505502632, -128.12507401300797, -129.71060822762783, -134.53859155226854, -134.73000777271366, -132.4609126111234, -132.29226702211295, -136.57800600993187, -151.1682586912211, -133.83977180579947, -130.0678401903246, -128.31600061089776, -127.08026292808452, -127.03493167845112, -127.45866969454404, -127.68676320629547, -129.09762856777132, -132.15364089986218, -134.04115428087206, -133.8779411464501, -132.0940499376788, -129.8350963346672, -128.85792307464442, -129.61110586568043, -130.96617607036728, -130.88154107532247, -129.28705567428938, -127.95609325559181, -127.50898840016848, -129.23559386268602, -134.04225947473645, -131.1340523000352, -130.92571209032178, -128.5602479879214, -125.6871345118046, -125.11912389362051, -126.24048123990843, -129.24535806163271, -132.5440886995646, -132.9954683362444, -136.12535515056248, -143.1618213572715, -133.94450536877093, -132.89376396921097, -129.6896132256777, -126.08767480217482, -124.78131242391572, -124.2630312563219, -124.11882131678357, -125.21905062996382, -128.20274801786485, -132.94546383836746, -134.2290453348339, -131.32176658377392, -129.71928378439375, -129.42446020016828, -129.8796130717054, -128.27635658130194, -128.42269621026605, -132.82075551623282, -136.1775161268704, -134.83166284300924, -130.91110156090878, -129.7226134122634, -131.44403452385663, -132.2830567724897, -129.7998097743775, -127.18084830701955, -125.85332351640282, -125.94019803617533, -127.12682941085392, -128.61695475350868, -129.7573076554893, -131.73105506979473, -136.52115876021065, -145.25392676654616, -154.40045789778497, -140.80592093742683, -133.8405262954971, -131.4216771987439, -132.78047100476175, -135.54634408756104, -135.95641648009197, -133.46076477633687, -133.3282158920459, -138.77983737457188, -146.53613685792283, -137.25006501914305, -131.0624241972309, -125.61996667947193, -122.73337965201776, -122.6992563957289, -125.0977045208799, -129.65788815938575, -133.85348282371456, -131.29842539900136, -132.32702770596177, -134.27326435823292, -129.1828971170441, -127.53331466556858, -128.04572023790135, -129.4051778201533, -129.12273514934617, -126.82476073177594, -126.7554523871324, -130.05646045486446, -133.12963431707558, -133.70846963996232, -133.5223055372282, -131.68011905188928, -129.97896879557206, -129.53502168992873, -131.03289102472633, -129.29673198034163, -126.46010756079349, -127.21270133997794, -131.69357233781957, -141.17552753342542, -136.92832494872553, -132.38809330970864, -129.99887465693874, -130.20986732760488, -133.24353656356416, -133.84431973429733, -131.92935389324722, -133.42639065281716, -151.35973915724958, -128.82271027063123, -124.41826711809475, -125.47774102219044, -133.53317624304682, -130.3583911258403, -124.85743487186735, -123.24232506273803, -123.76339290076822, -126.99586618548256, -134.3715325774083, -134.96014317682452, -135.35657690982578, -136.85181787996262, -129.80784607268754, -128.52967293150354, -131.41491565997063, -137.13644569463204, -142.48901007926804, -144.51871042193648, -145.09209018458304, -150.71861969534078, -135.16878599477513, -130.9569616252235, -131.03623501717556, -132.54770325374392, -134.4247607870267, -136.59539355594598, -137.52497886062497, -138.71558724297176, -138.41746910528656, -136.75402178489824, -137.21437189811726, -132.940815797596, -131.0676585481675, -131.5638283390021, -132.3066878366566, -131.2157643456185, -128.33466936681063, -125.23446374477857, -124.12297037494608, -125.29432052990711, -127.57046668571944, -128.26446586561138, -127.776321646176, -127.16152220808002, -127.35209371373928, -130.0907687167644, -135.6684518443326, -138.21315090732065, -152.4609447865921, -134.48178808548644, -130.01759392458277, -129.4730917772657, -130.3453988879159, -132.2639461793648, -134.90649021410974, -134.78473503413167, -132.669329445552, -130.12009501003504, -127.77708046934177, -126.77808648936565, -126.78420834383793, -126.71590271376998, -126.90819274472673, -127.22789333228658, -127.48929088218298, -128.97263443627816, -132.7769347586839, -139.69977867115097, -149.19674785010267, -152.17865615979935, -142.1370901485414, -137.74677040928768, -140.20479991167576, -141.07506969401268, -135.84160569739518, -137.802634000104, -137.61894173795017, -130.04495332145768, -128.41348087850938, -131.26771002653874, -141.2171291406108, -134.36825834126228, -129.38969535744138, -128.62711608009147, -130.46134580761253, -135.3957680861164, -133.6882063969853, -129.12944998676832, -127.3770015610652, -127.23452809472465, -129.0813257458891, -132.73323845111307, -133.57726679603837, -130.67114948878051, -127.23926945155878, -127.48248040997689, -134.37215283218256, -139.03530184710286, -133.01784867321197, -132.50157327394342, -133.73966978375861, -138.15023824330726, -143.39947510009046, -155.9002122867749, -138.7575097241884, -135.94465552586036, -135.45063865134813, -131.6361150865553, -133.65839942545674, -133.03202205011556, -130.69511024155904, -133.23961561594137, -130.9625727664657, -128.2153076780098, -129.50073724105584, -134.08546449654438, -142.98500668401434, -132.83058879553252, -127.92238330215369, -127.24529004289701, -129.66710715337135, -136.19331854126838, -136.57891579649348, -129.60805708964406, -125.83857397973244, -124.18455656206837, -125.82509641590299, -133.55683688476424, -142.68094701597934, -140.1839418614481, -149.88136548445934, -140.77509689187042, -137.3439060381786, -135.6073774197996, -134.59382376496316, -127.83802413343653, -123.4569105072813, -121.9162444877506, -122.56636607363548, -125.34405983355869, -130.93005959344578, -147.09119729373006, -133.1558767230698, -129.2034904394967, -131.72805963235714, -152.87033197938547, -134.36670548066212, -132.2186942690466, -129.05447011567892, -124.49607762043294, -122.90647848345458, -123.67046223611544, -124.71496206056527, -125.05820004559598, -125.85825841737775, -126.94981101712617, -127.15985773423732, -126.88855133984254, -126.98860611244501, -128.00773561683445, -131.0460962756032, -134.37880085402247, -131.30728603708317, -129.96168291858464, -133.53008250383613, -155.5540768314367, -138.36567815181735, -135.84263224308808, -136.0422912772776, -141.25333713549384, -146.58187309638276, -137.12326582685614, -136.9422025045508, -141.33436410845724, -136.35814017588535, -131.3728348484207, -129.5230521598017, -129.72181712332866, -130.69221607140526, -130.42489816045315, -128.5506576299286, -127.84934195614854, -130.16116489558974, -139.38179263679228, -133.5570474457268, -126.89291274222481, -124.47510236754111, -124.7402663253236, -128.53582197439843, -137.83349782972127, -133.07650712959463, -132.7316564601777, -135.5776014995986, -132.52765361345905, -129.33741630643516, -129.38656136633006, -131.58208588199494, -131.62006929528414, -128.86839835982119, -128.63477543108215, -132.5541484628382, -138.77322221928674, -137.99686851813948, -135.09984156358718, -133.83677615142577, -136.43883267057834, -136.27204172829119, -132.13441029060502, -132.7069277663301, -140.2458183872367, -141.55670152342304, -133.22348675328902, -131.60915130957335, -132.41073087902117, -132.89047906455585, -131.98319448150986, -132.42112942718467, -134.5587632714008, -134.70327853674715, -130.31895346886782, -126.34419365357417, -124.02623027387759, -122.93723644196761, -122.77935625545351, -123.74827789399163, -125.94459569490466, -128.08650089341668, -124.90172080007, -122.1703129181637, -122.40449683267107, -124.5380488139104, -126.81241159666806, -130.58631306824188, -140.2681581727165, -131.15261070817243, -127.31279000501118, -128.572482629686, -138.86784623426877, -132.9506017710833, -128.18866297039443, -129.03752988608738, -130.55442738921886, -127.86759171990248, -126.43104001391737, -127.20858230706257, -128.79872108858294, -129.82362063718205, -130.7794544040984, -131.03355884070035, -129.51427693590824, -127.86105487169847, -127.69472861806143, -126.99395981945997, -124.46450805175428, -123.0636928952014, -123.9251261901836, -126.67600206872643, -130.6178074159794, -137.6209434838156, -141.84610010477044, -131.66219781478054, -129.06985037405738, -131.1913037378464, -142.19909242700803, -138.31689786460888, -135.15212799812, -144.242448319401, -134.2250008614824, -132.46357048745276, -137.27282940880093, -135.67066277973896, -132.34310201367865, -132.94746139786696, -133.8153003609102, -134.61442293431713, -134.079348477098, -130.34588329095112, -126.85515797846071, -125.37791389056592, -125.2662950533064, -125.35373950145524, -126.19922569515971, -129.13063113227741, -133.3441633389782, -133.6546416639962, -130.2278697131692, -128.20879891221145, -128.76442722241464, -130.76381691919232, -131.61942174769985, -134.94575823027193, -151.22754853021496, -132.66579350926114, -127.84159721723547, -125.71199510700568, -124.74026138577364, -124.65298945605272, -125.59059276400369, -127.58620120374793, -131.52161098416053, -144.31071812393418, -135.03966223309084, -130.2238967846683, -129.61448413530178, -130.68891208152561, -133.46457869401786, -135.38720426559385, -131.50042122099643, -128.2110026163706, -126.72348819426463, -127.72106043587587, -133.4345269946623, -144.1150879910448, -134.89202011103873, -133.8505645371731, -133.42255338724183, -134.87629242273212, -137.35217498963223, -139.156378468693, -138.27443711979421, -133.8017355954073, -129.71798654204085, -127.63910504206754, -129.26107812138596, -137.00957808271923, -136.02353514190955, -134.80622118784115, -141.632067150959, -149.0901446827472, -139.05916172114587, -134.90164897945243, -131.25000766306627, -128.11499403116173, -127.49251434236486, -130.43745240754458, -135.51341724918993, -135.14539013526556, -132.09851422320313, -129.20811875778494, -127.7163044785978, -129.09416536303533, -130.39650144534005, -125.7284019523594, -123.35508352265761, -123.29661738895862, -124.0359525616217, -125.45872214665847, -128.31979843334165, -133.3578418093108, -138.3551528473419, -137.51247555116763, -136.45634768268326, -135.6904634745912, -136.75287509941, -131.55789255691434, -129.29764345151003, -129.52554863950806, -130.39241997392045, -131.53460253644502, -133.0419538685614, -135.14952422934797, -137.84363345667265, -138.00325862364463, -133.2010010366891, -129.56317599322315, -128.61129515391977, -128.96422328196607, -130.77120213064717, -130.51125411964426, -129.6604951406943, -133.37489035661247, -136.9623795293602, -135.11337995684502, -130.23490310186025, -126.06352306005451, -125.8041181124959, -130.54968258048117, -145.3264778754571, -135.903151113348, -135.36949207998117, -134.58896180587845, -133.8963201251977, -134.68004270895574, -138.2326599907626, -139.46725739643227, -137.87113178403519, -134.03635992558716, -129.5241632822, -128.36747606571785, -130.4422686523924, -136.22892063306654, -143.2583507852922, -141.73905035310892, -141.30794209898698, -148.30958467017194, -155.4840498795612, -142.3719162920506, -136.65570446659086, -134.05929813242602, -130.62710007053278, -127.63667236036198, -127.33126593763504, -128.26596937915997, -127.43752899446471, -125.99922601147557, -125.6024011671424, -126.81943961485075, -129.90872292943078, -130.16199440352614, -127.3403807691528, -126.74186941358062, -127.86276927563637, -128.48964107488726, -126.85846205149227, -126.08066016149274, -128.78659265282738, -137.6057054553821, -140.1361247805968, -134.1759636932037, -133.65306766276365, -136.34230898399298, -136.70499347710958, -136.74553810596439, -143.24395704993526, -138.8864022234338, -135.82214668837045, -133.5041265874072, -130.90484451058327, -130.5172835556203, -130.84785444009123, -129.74781186754254, -130.7352647968559, -134.40139823051663, -138.57033647203983, -139.83219059232346, -138.48988813062365, -137.73109034590473, -134.98944503335377, -136.82017260684816, -153.87812778816905, -139.95935450287433, -137.20192056857488, -136.477283336727, -135.87465861869998, -129.5009947250537, -126.07253484621948, -125.82694772041522, -127.87020642995758, -129.8397216002152, -128.81523409907055, -127.92197574772788, -127.83903444531546, -128.9274854374005, -132.489416702087, -140.33289489092834, -143.5671328879579, -133.06721578460656, -128.51833001179796, -126.65585921278418, -125.18233902769981, -123.8608730761642, -123.82677639482567, -125.61625264573551, -127.87964135489042, -128.03416234575604, -128.1480569799807, -128.81252853462811, -126.46041871771347, -124.25921713951702, -124.16480025921075, -126.05180346998773, -128.88832116398618, -130.23669825606828, -131.86123092111228, -138.0630021323617, -139.74524605544696, -132.85618990560488, -130.35918247697194, -131.43811219259229, -135.23548209576407, -133.8143493439313, -133.07256886053472, -135.8841465181784, -134.68986179616795, -129.14116432869895, -127.16341000153547, -127.1494431950965, -127.21601026141767, -128.19745572258893, -133.97030331651416, -135.03703132153075, -128.67375763075472, -129.2143579939396, -135.34880669536017, -139.5392912833014, -135.89714369674797, -135.98761202042527, -133.99748030898022, -130.23324501470947, -128.26833060776275, -128.70966560869792, -131.88189989766659, -134.4205113561923, -136.04979165223222, -139.91625623832138, -134.7541039717094, -133.06111278097487, -133.71783772523668, -134.2038791499006, -137.8864702670376, -136.06774133464535, -128.47319728906425, -127.79129850539613, -135.7685160744227, -132.9337522341328, -127.18410661439978, -128.19579279346556, -135.4847952052524, -140.16952856772525, -131.511901240472, -130.14071714233748, -131.93845710473593, -132.4998320434234, -130.70000442409588, -132.63419551253153, -141.3535122309366, -134.2902237642719, -129.77035916867175, -127.0480257492217, -125.71418288113495, -127.2348580791543, -132.43119653586305, -132.4722522344703, -132.33347598553004, -141.92894305807903, -133.1679436403757, -126.29232464345216, -123.92704357829547, -123.91236880010368, -125.72958908100965, -128.51648597680256, -128.15494941334603, -125.53137973074543, -124.89941703533475, -127.31030237591193, -131.28253114598866, -130.6340601862447, -129.00481440274572, -129.06675005372196, -130.85540297598047, -136.696220182427, -149.29447624289867, -136.73116844378066, -135.8912015758986, -139.37181131623066, -140.2426367985901, -135.78735207213248, -137.01913985062328, -141.73851424623427, -141.90803130879297, -140.97394186770725, -139.47783751622185, -135.63262649258536, -134.18076522907808, -132.87994196645596, -132.18221633949832, -133.33189621542832, -132.774959798471, -128.89128598684255, -126.44552023748346, -127.6279792567817, -133.45575740924002, -136.76243200740132, -135.59974573343803, -135.10647501061496, -131.56618454538463, -129.2085192461918, -127.2056076590058, -126.36314801681303, -129.04006810748243, -137.2796379357565, -138.58790429425773, -154.81731628275466, -135.9928482316798, -132.87797947231834, -133.04854801488045, -132.39582758485253, -130.29914740000106, -127.80756421508522, -125.70336965997649, -124.54728939091821, -124.28495595648143, -125.05916980505154, -127.32471714857418, -133.0838261227769, -136.5949328718823, -129.3875596157542, -128.37400929106752, -130.57398531378564, -134.71190479496505, -142.00491735221925, -140.99303672213816, -134.6117627632213, -134.24717067865978, -133.37247858681124, -133.26025244103545, -135.30301856043275, -134.6682815167232, -133.16945356051494, -134.114613758612, -134.79181892596634, -134.98775899051884, -137.7015577737468, -146.78164301464636, -146.04412771245023, -135.98614678040232, -131.6685597820763, -131.34652990925187, -134.87130531984232, -138.65920161248346, -134.7623278626678, -135.72767371311093, -141.52078891908408, -127.81314166192105, -124.88207716113821, -125.60137272311715, -129.07075845368743, -135.97312795083653, -145.08307019576358, -146.05306698966706, -135.85279976292682, -134.08605619699102, -134.37762565949183, -134.79153703136055, -142.86985103045606, -141.01329837879734, -136.9658647372742, -139.9637764048627, -140.72372140116207, -139.51366636689062, -136.47425776020927, -134.96106260096784, -134.6363411935791, -137.07653989352008, -145.62389613621022, -132.7360518005267, -129.15488629340257, -129.4357885646089, -132.64774974100095, -139.75999464970369, -138.770385125847, -136.13902001040248, -140.92272931485684, -142.7796246066468, -131.60087879399728, -127.40215064908745, -125.84275989898684, -126.69603647765575, -131.3152097254861, -144.87510239270082, -139.0393701445416, -141.9571131595175, -135.51669550190658, -127.84524297439744, -125.29302876704733, -126.55702400776497, -131.88732093077823, -133.70768856183335, -128.80275230905977, -127.468942863661, -129.75141061495663, -135.57451680229664, -136.56489051939454, -132.28292575663323, -129.5380111851425, -126.99699836136658, -126.14159016216067, -128.18953205257415, -128.69277733862663, -126.61501896130156, -127.67414116054874, -132.29517526810076, -137.78540180442366, -137.55722870873794, -138.0582083582497, -132.24824106358642, -128.32430746614804, -127.79458905784901, -130.23835243241527, -136.22432121324903, -138.48589612581907, -133.86799804411484, -133.62365918942797, -137.60346115539906, -135.47825040254855, -132.09075887268364, -129.9336558042438, -129.21424160918025, -130.7329016211909, -133.47404357391608, -134.17407163288132, -133.01474693422333, -131.8917893607841, -129.21319855428686, -127.47639043574836, -128.49946330466776, -131.01931548053267, -128.02640169115077, -126.33723782891676, -126.67455091851464, -126.89964586061764, -126.35830698710556, -127.4854251139625, -133.20041099613906, -143.08018465818196, -137.7597319843869, -133.62935948826416, -129.42420931005816, -128.6288586707673, -129.96486450641424, -132.70227495699447, -139.95106574358607, -131.51880486079153, -128.1525823713078, -129.02127588142613, -130.7512801489487, -131.7632722594093, -132.57525796956887, -132.22748652660263, -132.3118025331661, -135.43362844176656, -140.7338464327721, -138.71292921346355, -133.2691313629053, -132.08248347422506, -134.65543677497894, -134.05623040352972, -132.0319926525546, -131.78834386201453, -132.92425749981805, -135.84093747635833, -139.10846575167741, -141.30630922574252, -136.856307845199, -132.0366067122895, -130.47963029617844, -130.71206398122183, -131.09208113207546, -131.49215420601385, -132.23149614766058, -134.29716067690504, -138.5396115390439, -140.8508402494998, -137.44214252024864, -132.32021741182237, -128.1970988216412, -126.87876740912162, -128.10137818450002, -130.90069528131974, -132.50572431730905, -129.5563004466308, -127.3680470897473, -128.48313615452992, -134.23628268798615, -145.77791013233775, -135.76112049701632, -132.91163898168654, -133.2890514668762, -136.2890430379242, -138.9271392107912, -136.57554338788634, -132.63886627601642, -128.5456427297984, -127.27665227443961, -129.95448484202, -142.44732105657775, -134.49590612039907, -127.72840619157068, -125.64540585044627, -126.98479031146667, -131.62251042175666, -137.76626834704163, -138.11920600256056, -133.84773102045816, -131.98706413572336, -131.88532300338485, -131.29838762144078, -130.52335286044027, -130.1688325308169, -130.877358323427, -136.0238323343972, -141.57134124069964, -130.18929495137564, -127.15893863719351, -126.53384320182076, -127.26656277567714, -131.2047428860916, -149.38038878556304, -138.68607315496513, -142.3084100165932, -139.8207051794438, -132.16379301108478, -127.86258069188266, -127.20006212069849, -129.87350526866933, -136.4623997085685, -133.6705285323152, -130.13793720030125, -130.4285165946323, -127.98115455764666, -125.9883301361875, -126.81877111416608, -129.731613410685, -132.7244020560272, -133.95912192464556, -136.41366220332452, -137.40728639316455, -132.7293935603648, -129.79671836760687, -127.81542436483996, -127.34653312706538, -128.47657451702221, -130.29719074315608, -131.22168570813318, -130.91357849273044, -130.83759734760628, -131.5726894726696, -131.92058589951284, -128.93968621210885, -126.17322800504064, -124.55838129440099, -123.43413041134602, -123.76808913762443, -126.29591844611122, -131.04857718943765, -137.74293917724017, -143.35640743776824, -137.73195215879787, -132.9494978211167, -129.39901867709557, -127.23334649074401, -126.7425603131149, -128.08590674755777, -129.0510246480159, -126.05927376360052, -124.35543522630797, -124.96700292266357, -127.62692628900575, -133.5071740088858, -140.9755724702097, -130.10986110222746, -128.091760434452, -130.3648933368711, -135.3288086852055, -135.3248288880257, -131.9543555886135, -127.44789113409519, -124.67975173681072, -125.14946027519107, -128.02864878884867, -132.27489149922974, -139.60302107335593, -136.5851087261077, -129.88626318255933, -128.54667271457785, -131.18171326500382, -135.9474853916146, -136.97247561510508, -133.54914519253447, -130.43423325161757, -129.3608798647727, -131.25520596575896, -139.58370539522846, -140.13936967467566, -138.69307901550323, -139.57343017887246, -129.86297639275276, -126.83238872596029, -126.19443158090498, -127.42378213489827, -132.96945681074732, -142.82700287355422, -137.51670788570917, -135.42303491781797, -136.04696171996252, -134.2076897014687, -128.73949382895088, -127.25385618027487, -127.76112714342108, -126.85498855010508, -126.59876187092046, -127.85891645938455, -129.28325622786232, -131.1904039132838, -133.3439372074876, -136.41078511710856, -142.33268800665593, -131.18595446395142, -128.68733957718547, -131.25462637986982, -139.30959136994312, -139.43439782321977, -133.12588445239473, -130.90684665287168, -129.81420076109845, -129.7098977653642, -132.26466393503833, -136.20292277976193, -137.86081133288488, -138.9954014445237, -133.16840063619335, -131.559253031631, -134.6249247618291, -141.90665485614028, -136.27844401351132, -134.56549517253126, -137.9586532068894, -136.73999611002185, -130.59423750928292, -127.8094513181745, -128.71108197036202, -133.10969086395528, -135.10388593615605, -130.01241014517572, -127.37739311594058, -127.06093248443605, -128.33116882248916, -132.21383938939698, -137.00549160874576, -131.84782014257087, -129.06581757996608, -127.93413896036581, -128.08320528067674, -128.49428492026453, -129.0534504683654, -130.25093492297285, -129.3278350587986, -128.43603239703788, -130.40117526001208, -133.1996004292252, -131.66277063350162, -130.09026578562296, -131.49011233321102, -139.30098529470771, -138.9623834819106, -130.07863465769034, -127.69841404551676, -128.82365701609385, -134.23266317017325, -143.70607612555813, -134.14188793695388, -131.3137301758001, -131.8671193875728, -135.76709429642153, -154.90372327289737, -137.35690182289258, -133.6220992462147, -133.4856439517186, -137.49465073958658, -137.08509937984886, -132.70390635043918, -132.65631944073112, -134.17650658609367, -135.96387070568943, -137.77299029727888, -137.19716467897732, -134.08719663673128, -130.29432174937492, -127.66955969307054, -127.84802000190848, -131.30921614199, -134.82699230442284, -141.9294430883929, -138.42756675797628, -132.65280494198674, -127.48643853914078, -123.02480194662202, -121.99617797199488, -124.31107107595473, -128.70037732205407, -130.77632561674181, -131.53334047024265, -133.215045422695, -130.61680758024212, -128.22242121489762, -128.66242870883946, -128.99208847255355, -127.71567610907944, -128.16191142771052, -133.15597024640175, -133.8411538699499, -128.49532742149898, -127.17330534097721, -127.86343060710892, -129.28061413080658, -128.77170629899115, -127.90843879612206, -129.24243310297666, -129.95915934268797, -129.79220481070354, -133.58563669057924, -140.08578889276106, -139.69057850509483, -134.6307089440079, -132.0339921356036, -132.12816396578117, -133.66868247591822, -135.54383235457087, -136.32546447571028, -133.61693301004857, -130.76779417857293, -127.27800091134151, -125.89599665985315, -127.90132924668345, -131.00658120730355, -129.0207043104167, -127.49730108740744, -128.8050105103249, -133.31682590565399, -140.56056449077357, -135.60217976557033, -129.3985687034139, -125.55170551217802, -124.22791372072176, -125.00607470674649, -125.87833038288596, -124.61666287108082, -123.23446539883429, -123.65323290535316, -125.45186318714521, -126.69183347467545, -127.25025401825926, -128.70666672101598, -131.34519346121678, -133.24919328702333, -132.8531739961499, -131.3199288040173, -132.04004072859973, -135.9343501151219, -131.1702867504857, -128.54968720242073, -129.85994418593637, -133.4688431899259, -135.16775575879106, -133.10997811063547, -132.18777182173554, -132.07167699770406, -130.66898150571222, -131.4776462076446, -132.54902844640858, -135.0762545184414, -145.19359017321275]} ("FreqDomainGraph"), "x0"=w3, "dx"=w2, "magnitude"=w1) -> (→"FreqDomainGraph":cluster{"x0":dbl, "dx":dbl, "magnitude":dbl[]})
  n34 = Bundle By Name(cluster=T9 {"Channel"="", "Calculated frequency"=0.0, "Calculated amplitude"=0.0, "SNR"=0.0, "THD+N"=0.0, "THD"=0.0, "Dynamic range"=0.0, "Gain error"=0.0, "SFDR"=0.0, "t0"=0.0, "dt"=0.0, "Time domain"=[], "f0"=0.0, "df"=0.0, "Spectrum"=[], "Sample rate"=0} ("Measurement Results"), "f0"=w3, "df"=w2, "Spectrum"=w1, "Gain error"=w24, "Dynamic range"=w23, "SFDR"=w22, "Calculated frequency"=w21, "Calculated amplitude"=w20, "SNR"=w19, "THD+N"=w18, "THD"=w17, "t0"=0.0 ("Wfm t0"), "dt"=w15, "Time domain"=w14) -> (→"output cluster":T9)
